vi "19.0422.vi"() -> ()   [LabVIEW 2015]
uses:
  Control 1.ctl
  <vilib>/DAQmx/read.llb/DAQmx Read (Digital 1D Bool 1Chan 1Samp).vi
  <vilib>/DAQmx/write.llb/DAQmx Write (Digital Bool 1Line 1Point).vi
  <vilib>/DAQmx/write.llb/DAQmx Write (Digital 1D Bool 1Chan 1Samp).vi
  <vilib>/DAQmx/create/channels.llb/DAQmx Create Channel (DO-Digital Output).vi
  <vilib>/DAQmx/miscellaneous.llb/DAQmx Fill In Error Info.vi
panel:
  in  "data":bool[](array[boolean])
  in  "Adress":bool[](array[boolean])
  in  "Считать данные":bool
  in  "Записать данные":bool
  out "data 2":bool[](array[boolean])
  out "Enum":T1
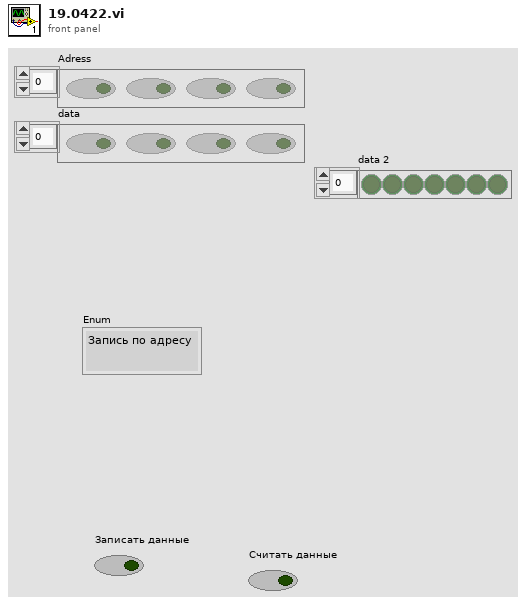
[diagram p1: front panel]
types:
  T1 = typedef "Control 1.ctl" = enum16{"Запись по адресу", "Чтение по адресу", "Тактирование ", "Ожидание"}
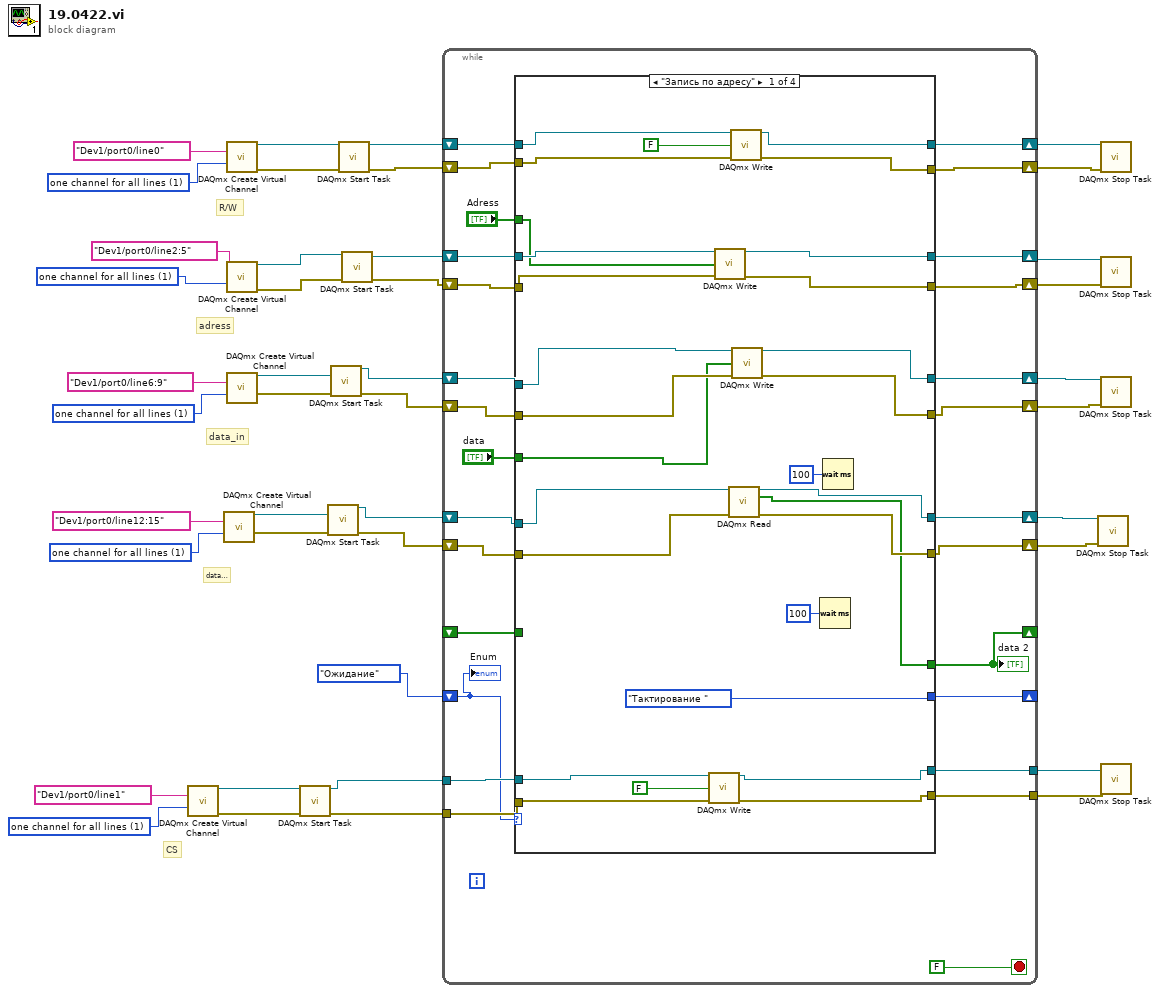
[diagram p0: block diagram]
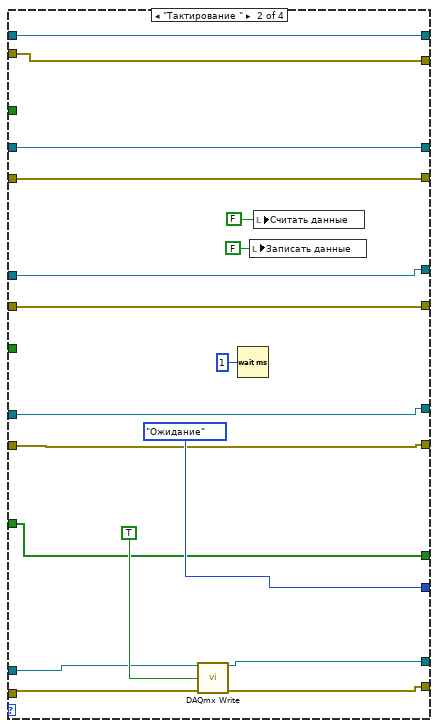
[diagram p2: hidden frame]
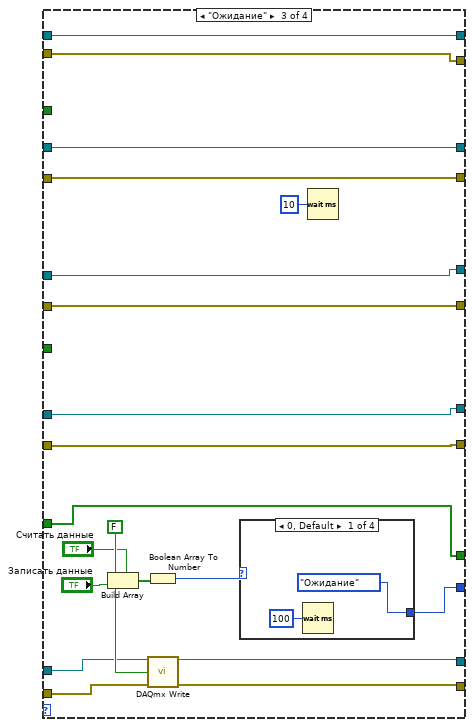
[diagram p3: hidden frame]
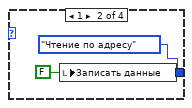
[diagram p4: hidden frame]
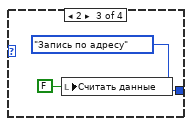
[diagram p5: hidden frame]
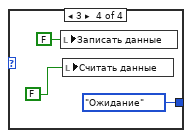
[diagram p6: hidden frame]
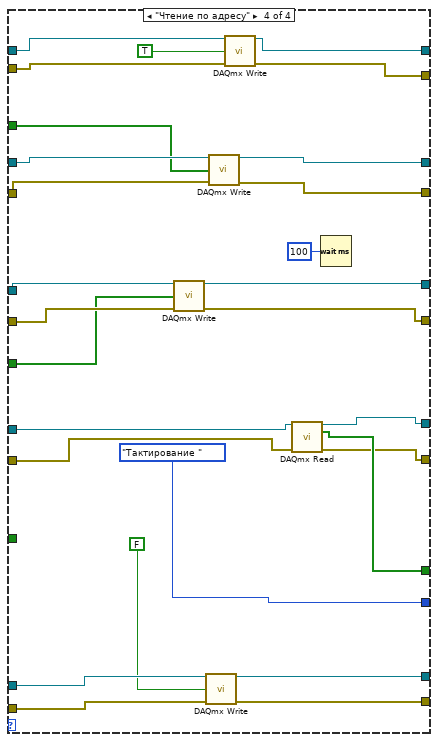
[diagram p7: hidden frame]
diagram:
  w2 = 1 items=["one channel for each line", "one channel for all lines"] ("line grouping")
  w16 = 1 items=["one channel for each line", "one channel for all lines"] ("line grouping")
  w24 = 1 items=["one channel for each line", "one channel for all lines"] ("line grouping")
  w33 = 1 items=["one channel for each line", "one channel for all lines"] ("line grouping")
  w35 = 1 items=["one channel for each line", "one channel for all lines"] ("line grouping")
  # "data out"
  # "CS"
  # "data_in"
  # "adress"
  # "R/W"
  n1 = call-poly <vilib>:"DAQmx Create Virtual Channel.vi"("lines"=tag "Dev1/port0/line1", "line grouping"=w16) -> ("task out"=w15:refnum<k21>, "error out"=w14:errorcluster)  [unwired: 12 in]
  n2 = call-poly <vilib>:"DAQmx Create Virtual Channel.vi"("lines"=tag "Dev1/port0/line12:15", "line grouping"=w2) -> ("task out"=w5:refnum<k21>, "error out"=w6:errorcluster)  [unwired: 12 in]
  n3 = call-poly <vilib>:"DAQmx Create Virtual Channel.vi"("lines"=tag "Dev1/port0/line0", "line grouping"=w35) -> ("task out"=w36:refnum<k21>, "error out"=w37:errorcluster)  [unwired: 12 in]
  n4 = call-poly <vilib>:"DAQmx Create Virtual Channel.vi"("lines"=tag "Dev1/port0/line2:5", "line grouping"=w33) -> ("task out"=w32:refnum<k21>, "error out"=w31:errorcluster)  [unwired: 12 in]
  n5 = call-poly <vilib>:"DAQmx Create Virtual Channel.vi"("lines"=tag "Dev1/port0/line6:9", "line grouping"=w24) -> ("task out"=w21:refnum<k21>, "error out"=w20:errorcluster)  [unwired: 12 in]
  n6 = call <vilib>:"DAQmx Start Task.vi"("task/channels in"=w15, "error in"=w14) -> ("task out"=w13:refnum<k21>, "error out"=w12:errorcluster)  [unwired: 12 in]
  n7 = call <vilib>:"DAQmx Start Task.vi"("task/channels in"=w5, "error in"=w6) -> ("task out"=w7:refnum<k21>, "error out"=w8:errorcluster)  [unwired: 12 in]
  n8 = call <vilib>:"DAQmx Start Task.vi"("task/channels in"=w21, "error in"=w20) -> ("task out"=w19:refnum<k21>, "error out"=w18:errorcluster)  [unwired: 12 in]
  n9 = call <vilib>:"DAQmx Start Task.vi"("task/channels in"=w36, "error in"=w37) -> ("task out"=w38:refnum<k21>, "error out"=w39:errorcluster)  [unwired: 12 in]
  n10 = call <vilib>:"DAQmx Start Task.vi"("task/channels in"=w32, "error in"=w31) -> ("task out"=w30:refnum<k21>, "error out"=w29:errorcluster)  [unwired: 12 in]
  n11 = while {
    shift-right: [w68] -> w41
    shift-left: w39 -> [w66]
    shift-right: [w67] -> w40
    shift-left: w38 -> [w65]
    shift-right: [w56] -> w27
    shift-left: w29 -> [w63]
    shift-right: [w60] -> w23
    shift-left: w19 -> [w58]
    shift-right: [w59] -> w22
    shift-left: w18 -> [w57]
    shift-right: [w62] -> w28
    shift-left: w30 -> [w64]
    tunnel: w13 -> [w55]
    tunnel: w12 -> [w54]
    tunnel: [w53] -> w11
    tunnel: [w52] -> w10
    shift-right: [w51] -> _
    shift-left: Control_1."Ожидание" ("Enum") -> [w49]
    shift-right: [w50] -> _
    shift-left: _ -> [w42]
    shift-right: [w43] -> w3
    shift-left: w7 -> [w45]
    shift-right: [w44] -> w4
    shift-left: w8 -> [w46]
    stop <- FALSE stop-if-true
    n12 = case shown="\"Запись по адресу\"" w49 {
      tunnel: [w85 w105 w125 w163] -> w68
      tunnel: [w84 w104 w124 w162] -> w67
      tunnel: w66 -> [w86 w105 w125 w164]
      tunnel: w65 -> [w87 w104 w124 w165]
      tunnel: w64 -> [w96 w106 w126 w170]
      tunnel: w63 -> [w95 w107 w127 w169]
      tunnel: [w94 w106 w126 w168] -> w62
      tunnel: [w93 w107 w127 w167] -> w56
      tunnel: [w92 w108 w128 w159] -> w60
      tunnel: [w91 w109 w129 w158] -> w59
      tunnel: w58 -> [w90 w108 w128 w161]
      tunnel: w57 -> [w89 w109 w129 w160]
      tunnel: [w69 w99 w117 w149] -> w50
      tunnel: w55 -> [w80 w113 w133 w157]
      tunnel: w54 -> [w79 w112 w132 w156]
      tunnel: [w82 w111 w131 w154] -> w53
      tunnel: [w81 w110 w130 w153] -> w52
      tunnel: [Control_1."Тактирование " ("Enum") Control_1."Ожидание" ("Enum") w119 Control_1."Тактирование " ("Enum")] -> w51
      tunnel: "Adress" -> [w76 _ _ w150]
      tunnel: "data" -> [w75 _ _ w144]
      tunnel: [w71 w98 w116 w148] -> w43
      tunnel: [w72 w97 w115 w147] -> w44
      tunnel: w45 -> [w70 w98 w116 w146]
      tunnel: w46 -> [w73 w97 w115 w145]
      tunnel: w42 -> [_ w99 w117 _]
      frame "Запись по адресу" {
        n13 = call-poly <vilib>:"DAQmx Write.vi"("task/channels in"=w80, "data"=FALSE, "error in"=w79) -> ("task out"=w82:refnum<k21>, "error out"=w81:errorcluster)  [unwired: 10 in, 1 out]
        n14 = call-poly <vilib>:"DAQmx Write.vi"("task/channels in"=w96, "data"=w76, "error in"=w95) -> ("task out"=w94:refnum<k21>, "error out"=w93:errorcluster)  [unwired: 10 in, 1 out]
        n15 = call-poly <vilib>:"DAQmx Read.vi"("task/channels in"=w70, "error in"=w73) -> ("task out"=w71:refnum<k21>, "data"=w69:bool[], "error out"=w72:errorcluster)  [unwired: 11 in]
        n16 = call-poly <vilib>:"DAQmx Write.vi"("task/channels in"=w87, "data"=FALSE, "error in"=w86) -> ("task out"=w84:refnum<k21>, "error out"=w85:errorcluster)  [unwired: 10 in, 1 out]
        n17 = call-poly <vilib>:"DAQmx Write.vi"("task/channels in"=w90, "data"=w75, "error in"=w89) -> ("task out"=w92:refnum<k21>, "error out"=w91:errorcluster)  [unwired: 10 in, 1 out]
        n18 = Wait (ms)(milliseconds to wait=u32 100) -> ()  [unwired: 1 out]
        n19 = Wait (ms)(milliseconds to wait=u32 100) -> ()  [unwired: 1 out]
      }
      frame "Тактирование " {
        n20 = call-poly <vilib>:"DAQmx Write.vi"("task/channels in"=w113, "data"=TRUE, "error in"=w112) -> ("task out"=w111:refnum<k21>, "error out"=w110:errorcluster)  [unwired: 10 in, 1 out]
        n21 = Wait (ms)(milliseconds to wait=u32 1) -> ()  [unwired: 1 out]
        n22 = local write "Записать данные"(FALSE ("Записать данные")) -> ()
        n23 = local write "Считать данные"(FALSE ("Записать данные")) -> ()
      }
      frame "Ожидание" {
        n24 = Build Array("Считать данные", "Записать данные") -> (w121:bool[])
        n25 = Boolean Array To Number(Boolean array=w121) -> (number=w120:u32)
        n26 = call-poly <vilib>:"DAQmx Write.vi"("task/channels in"=w133, "data"=FALSE, "error in"=w132) -> ("task out"=w131:refnum<k21>, "error out"=w130:errorcluster)  [unwired: 10 in, 1 out]
        n27 = case shown="0, Default" w120 {
          tunnel: [Control_1."Ожидание" ("Enum") Control_1."Чтение по адресу" ("Enum") Control_1."Запись по адресу" ("Enum") Control_1."Ожидание" ("Enum")] -> w119
          frame 0, Default {
            n28 = Wait (ms)(milliseconds to wait=u32 100) -> ()  [unwired: 1 out]
          }
          frame 1 {
            n29 = local write "Записать данные"(FALSE ("Записать данные")) -> ()
          }
          frame 2 {
            n30 = local write "Считать данные"(FALSE ("Считать данные")) -> ()
          }
          frame 3 {
            n31 = local write "Записать данные"(FALSE ("Записать данные")) -> ()
            n32 = local write "Считать данные"(FALSE ("Считать данные")) -> ()
          }
        }
        n33 = Wait (ms)(milliseconds to wait=u32 10) -> ()  [unwired: 1 out]
      }
      frame "Чтение по адресу" {
        n34 = call-poly <vilib>:"DAQmx Write.vi"("task/channels in"=w161, "data"=w144, "error in"=w160) -> ("task out"=w159:refnum<k21>, "error out"=w158:errorcluster)  [unwired: 10 in, 1 out]
        n35 = call-poly <vilib>:"DAQmx Write.vi"("task/channels in"=w157, "data"=FALSE, "error in"=w156) -> ("task out"=w154:refnum<k21>, "error out"=w153:errorcluster)  [unwired: 10 in, 1 out]
        n36 = call-poly <vilib>:"DAQmx Write.vi"("task/channels in"=w170, "data"=w150, "error in"=w169) -> ("task out"=w168:refnum<k21>, "error out"=w167:errorcluster)  [unwired: 10 in, 1 out]
        n37 = call-poly <vilib>:"DAQmx Write.vi"("task/channels in"=w165, "data"=TRUE, "error in"=w164) -> ("task out"=w162:refnum<k21>, "error out"=w163:errorcluster)  [unwired: 10 in, 1 out]
        n38 = call-poly <vilib>:"DAQmx Read.vi"("task/channels in"=w146, "error in"=w145) -> ("task out"=w148:refnum<k21>, "data"=w149:bool[], "error out"=w147:errorcluster)  [unwired: 11 in]
        n39 = Wait (ms)(milliseconds to wait=u32 100) -> ()  [unwired: 1 out]
      }
    }
    "data 2" <- w50
    "Enum" <- w49
  }
  n40 = call <vilib>:"DAQmx Stop Task.vi"("task/channels in"=w3, "error in"=w4) -> ()  [unwired: 12 in, 2 out]
  n41 = call <vilib>:"DAQmx Stop Task.vi"("task/channels in"=w40, "error in"=w41) -> ()  [unwired: 12 in, 2 out]
  n42 = call <vilib>:"DAQmx Stop Task.vi"("task/channels in"=w28, "error in"=w27) -> ()  [unwired: 12 in, 2 out]
  n43 = call <vilib>:"DAQmx Stop Task.vi"("task/channels in"=w23, "error in"=w22) -> ()  [unwired: 12 in, 2 out]
  n44 = call <vilib>:"DAQmx Stop Task.vi"("task/channels in"=w11, "error in"=w10) -> ()  [unwired: 12 in, 2 out]
